vi "Find Asset.vi"(8 "error in (no error)":errorcluster, 10 "Serial Number":string="1234", 11 "Part Number":string="B0CG1KL3RC") -> (0 "error out":errorcluster, 2 "Properties":string[][](array[string]), 3 "Asset ID":string)   [LabVIEW 2024]
uses:
  SupportVIs/NI Skyline Configuration HTTP.lvclass/NI Skyline Configuration HTTP.ctl
  57c89dda-b992-40f1-af52-fb23adf69676.vi
  aee58dd2-821e-4a5f-8d8b-37a18e53902b.vi
  SupportVIs/Read Server URL.vi
  SupportVIs/Next JSON Value.vi
  SupportVIs/String Subset.vi
  SupportVIs/Advance past next JSON Value (inlined COPY).vi
  SupportVIs/Advance past whitespace.vi
  SupportVIs/Advance past String.vi
  SupportVIs/Advance past Number.vi
  SupportVIs/Advance past Line Ending.vi
  SupportVIs/Open Configuration HTTP Auto.vi
  SupportVIs/POSTBuffer.vi
  SupportVIs/Parse Full Path or Item Name.vi
  SupportVIs/Advance past Array.vi
  SupportVIs/Advance past Object.vi
  SupportVIs/Error Cluster From Code.vi
  SupportVIs/Find Item Locations by Path.vi
  SupportVIs/JSON text to Variant.vi
  SupportVIs/JSONtext LVClass Serializer.lvclass
  SupportVIs/NI Skyline Configuration HTTP.lvclass
  SupportVIs/LabVIEWHTTPClient.lvlib
  SupportVIs/JSONtext.lvlib
panel:
  out "body":string
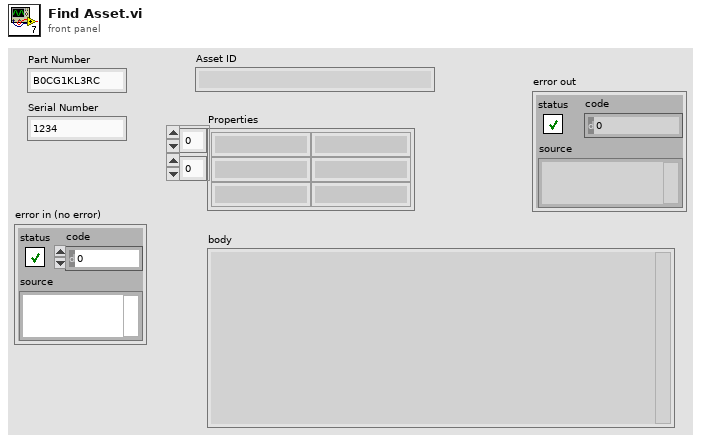
[diagram p1: front panel]
types:
  T1 = typedef "LabVIEWHTTPClient.lvlib/ClientHandle.ctl" = refnum<k1>
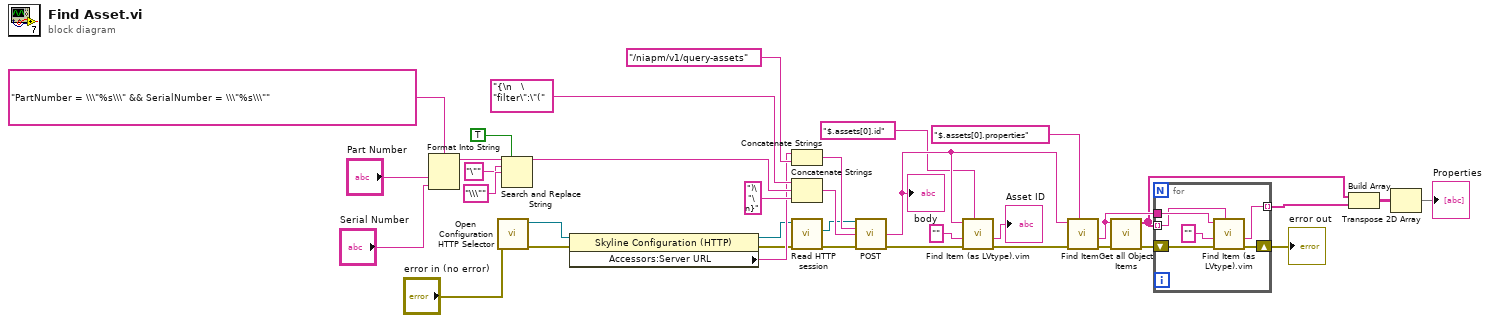
[diagram p0: block diagram]
diagram:
  n1 = Format Into String(format string="PartNumber = \\\"%s\\\" && SerialNumber = \\\"%s\\\"", "Part Number", "Serial Number") -> (resulting string=w32:string)  [unwired: 2 in, 1 out]
  n2 = call-poly "Open Configuration HTTP Selector.vi"("error in (no error)"="error in (no error)") -> ("error out"=w19:errorcluster, "configuration"=w17:refnum<class "NI Skyline Configuration HTTP.lvclass">)  [unwired: 9 in]
  n3 = Search and Replace String(replace all?=TRUE ("replace all? (F)"), input string=w32, search string="\"", replace string="\\\"" ("replace string (\"\")")) -> (result string=w35:string)  [unwired: 4 in, 3 out]
  n4 = property on="Property Node" class="Skyline Configuration (HTTP)"(reference=w17, error in=w19) -> (reference out=w22:refnum<class "NI Skyline Configuration HTTP.lvclass">, error out=w18:errorcluster, "Accessors:Server URL"=w23:string)
  n5 = Concatenate Strings(w23, "/niapm/v1/query-assets" ("url")) -> (w25:string)
  n6 = Concatenate Strings("{\n   \"filter\":\"(", w35, ")\"\n}") -> (w31:string)
  n7 = call "Read HTTP session.vi"("error in (no error)"=w18, "HTTP configuration in"=w22) -> ("error out"=w21:errorcluster, "http session"=w20:T1)  [unwired: 7 in, 1 out]
  n8 = call-poly "POST.vi"("client handle"=w20, "url"=w25, "buffer"=w31, "error in (no error)"=w21) -> ("body"=w12:string, "error out"=w8:errorcluster)  [unwired: 8 in, 2 out]
  "body" <- w12
  n9 = call "Find Item (as LVtype).vim"("$Path or Item Name"="$.assets[0].id", "error in (no error)"=w8, "Data Type and Default Value"="", "JSON"=w12) -> ("error out"=w9:errorcluster, "Data"=→"Asset ID":string)  [unwired: 4 in, 2 out]
  n10 = call "Find Item.vi"("$Path or Item Name"="$.assets[0].properties", "error in (no error)"=w9, "JSON"=w12) -> ("error out"=w6:errorcluster, "<JSON>"=w15:string)  [unwired: 5 in, 2 out]
  n11 = call "Get all Object Items.vi"("error in (no error)"=w6, "JSON"=w15) -> ("error out"=w5:errorcluster, "Item Names"=w14:string[])  [unwired: 6 in, 2 out]
  n12 = for {
    tunnel: w14 -> [w41] mode=indexing
    tunnel: w15 -> [w42]
    tunnel: [w39] -> w13 mode=indexing
    shift-right: [w37] -> w4
    shift-left: w5 -> [w38]
    n13 = call "Find Item (as LVtype).vim"("$Path or Item Name"=w41, "error in (no error)"=w38, "Data Type and Default Value"="", "JSON"=w42) -> ("error out"=w37:errorcluster, "Data"=w39:string)  [unwired: 4 in, 2 out]
  }
  "error out" <- w4
  n14 = Build Array(w14, w13) -> (w3:string[][])
  n15 = Transpose 2D Array(2D array=w3) -> (transposed array=→"Properties":string[][])
